vi "McPherson Max Errors.vi"(1 "stop":bool, 2 "error":bool) -> (0 "Cont?":bool)   [LabVIEW 2025]
doc: "Author: Scott Hannahs <sth@magnet.fsu.edu>\n\nThis software is licensed for use under the “MIT License\"\nCopyright (c) 2025 Scott Hannahs, sth@sth@magnet.sthnet.net\n\nPermission is hereby granted, free of charge, to any person obtaining a copy of this software and associated documentation files (the \"Software\"), to deal in the Software without restriction, including without limitation the rights to use, copy, modify, merge, publish, distribute, sublicense, and/or sell copies of the Software, and to permit persons to whom the Software is furnished to do so, subject to the following conditions: The above copyright notice and this permission notice shall be included in all copies or substantial portions of the Software.\n\nTHE SOFTWARE IS PROVIDED \"AS IS\", WITHOUT WARRANTY OF ANY KIND, EXPRESS OR IMPLIED, INCLUDING BUT NOT LIMITED TO THE WARRANTIES OF MERCHANTABILITY, FITNESS FOR A PARTICULAR PURPOSE AND NONINFRINGEMENT. IN NO EVENT SHALL THE AUTHORS OR COPYRIGHT HOLDERS BE LIABLE FOR ANY CLAIM, DAMAGES OR OTHER LIABILITY, WHETHER IN AN ACTION OF CONTRACT, TORT OR OTHERWISE, ARISING FROM, OUT OF OR IN CONNECTION WITH THE SOFTWARE OR THE USE OR OTHER DEALINGS IN THE SOFTWARE."
uses:
  Globals and TypeDefs/gSpectrometer.vi
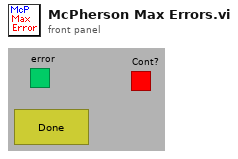
[diagram p1: front panel]
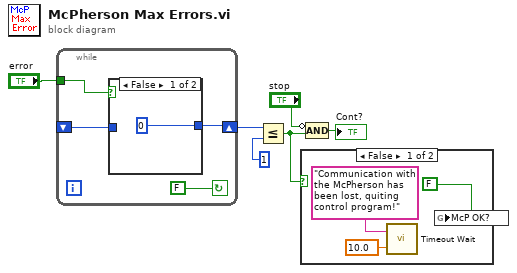
[diagram p0: block diagram]
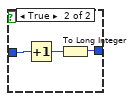
[diagram p2: hidden frame]
diagram:
  n1 = while {
    tunnel: "error" -> [w10]
    shift-left: _ -> [w8]
    shift-right: [w9] -> w5
    stop <- FALSE continue-if-true
    n2 = case shown="False" w10 {
      tunnel: [0 w12] -> w9
      tunnel: w8 -> [_ w14]
      frame False {
      }
      frame True {
        n3 = Increment(x=w14) -> (x+1=w13:i32)
        n4 = To Long Integer(number=w13) -> (32bit integer=w12:i32)
      }
    }
  }
  n5 = Less Or Equal?(x=w5, y=1) -> (x <= y?=w3:bool)
  n6 = case shown="False" w3 {
    frame False {
      n7 = call "Timeout Wait.vi"("Seconds to timeout"=10.0, "Message"="Communication with the McPherson has been lost, quiting control program!" ("message")) -> ()
      n8 = global write "gSpectrometer.vi" "McP OK?"(FALSE ("McP OK?")) -> ()
    }
    frame True {
    }
  }
  n9 = Compound Arithmetic op=AND(invert "stop", w3) -> (→"Cont?":bool)
